vi "DMSP_add_NaOH_BM.vi"(6 "COM Port":refnum<visa-resource-name>="COM4", 7 "Pump Parameters":T1={"Speed 1"="100", "Speed 2"="250", "Speed 3"="350", "Speed 4"="250", "UW/Sample"="5", "Sparge"="2", "Std"="4", "Waste"="15", "Air"="14", "Milli-Q"="1", "H2SO4"="6", "NaOH"="3", "Catalyst"="7", "Cell (H+ side)"="8", "Cell (sample side)"="9", "NaCl"="11"}, 8 "NaOH Vol (mL)":dbl=3.0, 9 "step to ml":dbl=1920.0, 10 "Total Vol. (mL)":dbl=10.0, 11 "Sample Vol. (mL)":dbl=10.0) -> ()   [LabVIEW 2021]
panel:
  out "Full Command":string="o4A0V5000o1P14400o4D14400o1P33600o4D9600o2D24000o5P9600o2D9600o6P33600o4D33600"
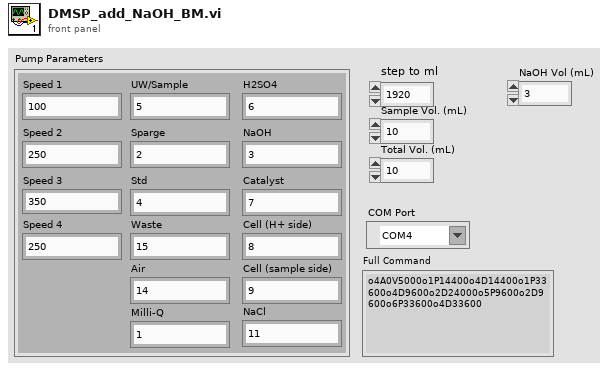
[diagram p1: front panel]
types:
  T1 = cluster{"Speed 1":string, "Speed 2":string, "Speed 3":string, "Speed 4":string, "UW/Sample":string, "Sparge":string, "Std":string, "Waste":string, "Air":string, "Milli-Q":string, "H2SO4":string, "NaOH":string, "Catalyst":string, "Cell (H+ side)":string, "Cell (sample side)":string, "NaCl":string}
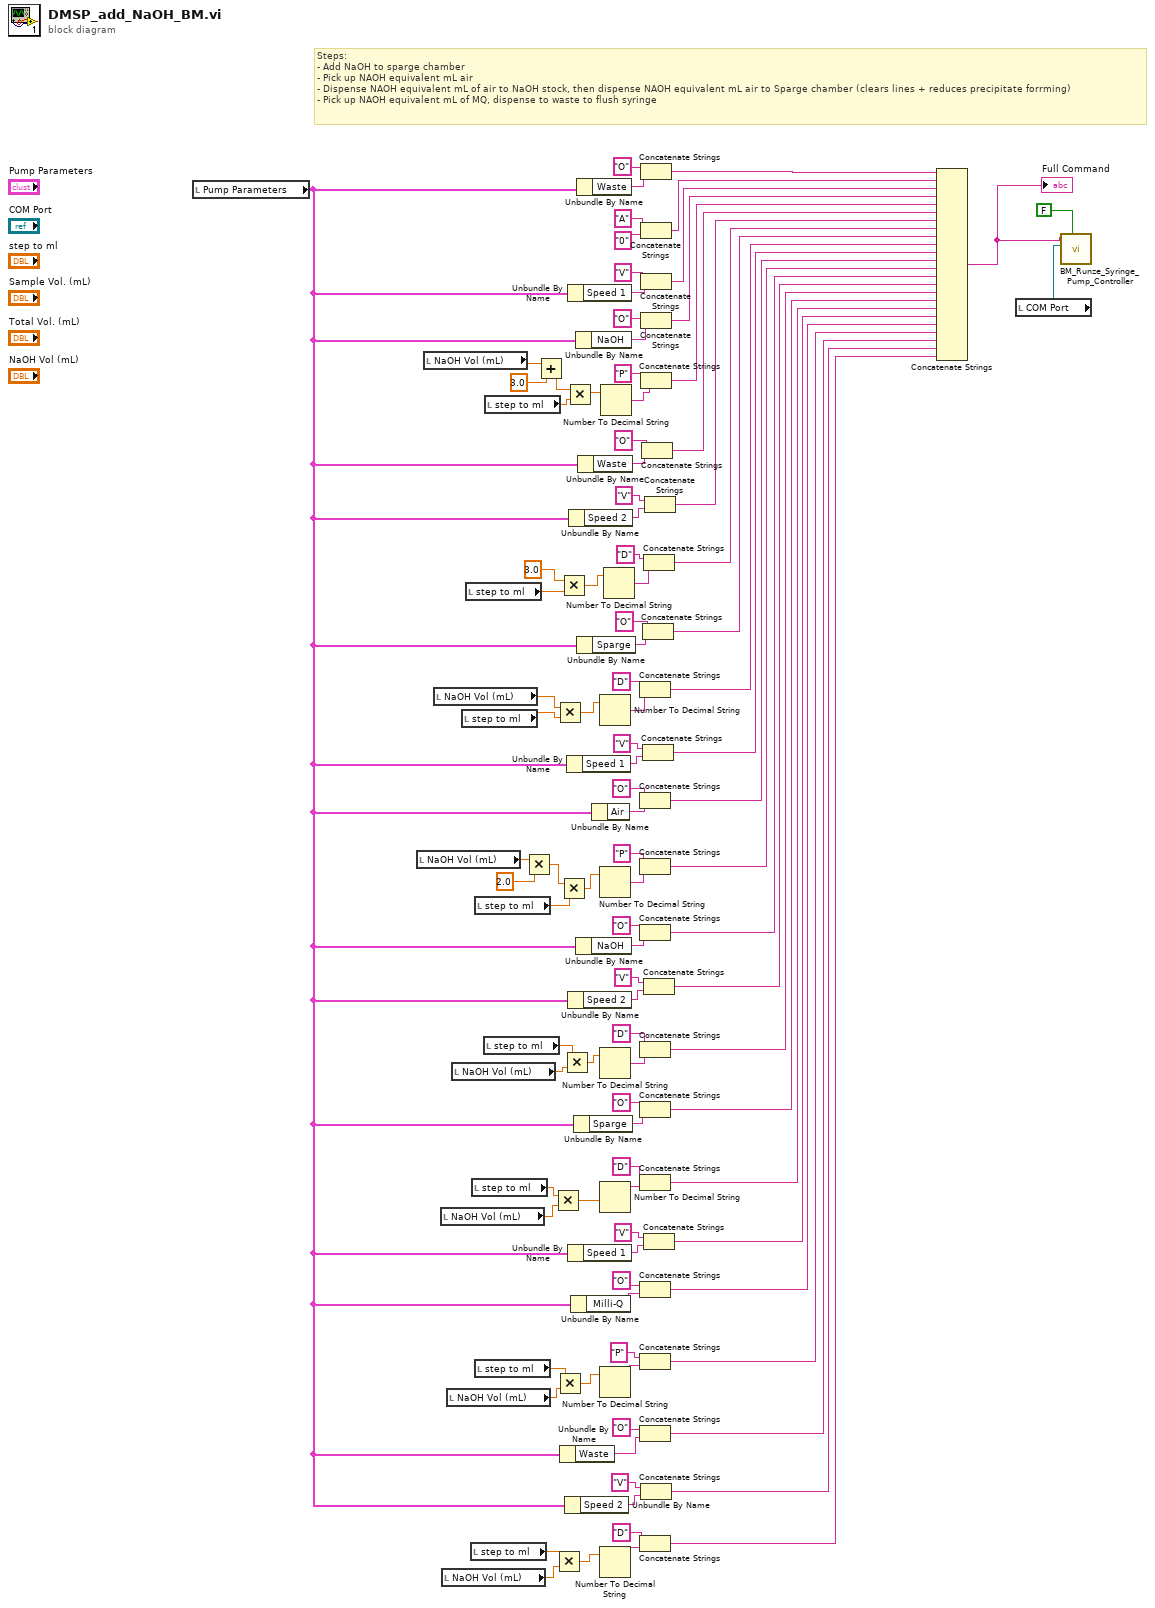
[diagram p0: block diagram]
diagram:
  # "Steps:\n- Add NaOH to sparge chamber\n- Pick up NAOH equivalent mL air \n- Dispense NAOH equivalent mL of air to NaOH stock, then dispense NAOH equivalent mL air to Sparge chamber (clears lines + reduces precipitate forrming)\n- Pick up NAOH equivalent mL of MQ, dispense to waste to flush syringe"
  n1 = local read "Pump Parameters"() -> (w10:T1)
  n2 = local read "NaOH Vol (mL)"() -> (w22:dbl)
  n3 = local read "NaOH Vol (mL)"() -> (w13:dbl)
  n4 = local read "NaOH Vol (mL)"() -> (w23:dbl)
  n5 = local read "NaOH Vol (mL)"() -> (w17:dbl)
  n6 = local read "NaOH Vol (mL)"() -> (w19:dbl)
  n7 = local read "NaOH Vol (mL)"() -> (w18:dbl)
  n8 = local read "NaOH Vol (mL)"() -> (w16:dbl)
  n9 = local read "step to ml"() -> (w71:dbl)
  n10 = local read "step to ml"() -> (w8:dbl)
  n11 = local read "step to ml"() -> (w60:dbl)
  n12 = local read "step to ml"() -> (w85:dbl)
  n13 = local read "step to ml"() -> (w86:dbl)
  n14 = local read "step to ml"() -> (w84:dbl)
  n15 = local read "step to ml"() -> (w87:dbl)
  n16 = local read "step to ml"() -> (w88:dbl)
  n17 = Multiply(x=w22, y=2.0) -> (x*y=w20:dbl)
  n18 = Add(x=w13, y=3.0) -> (x+y=w15:dbl)
  n19 = Multiply(x=w85, y=w17) -> (x*y=w103:dbl)
  n20 = Multiply(x=w60, y=w19) -> (x*y=w61:dbl)
  n21 = Multiply(x=w23, y=w71) -> (x*y=w72:dbl)
  n22 = Multiply(x=w84, y=w18) -> (x*y=w102:dbl)
  n23 = Multiply(x=3.0, y=w8) -> (x*y=w7:dbl)
  n24 = Multiply(x=w20, y=w86) -> (x*y=w101:dbl)
  n25 = Unbundle By Name(w10) -> ("Waste"=w75:string)
  n26 = Multiply(x=w87, y=w16) -> (x*y=w104:dbl)
  n27 = Multiply(x=w15, y=w88) -> (x*y=w100:dbl)
  n28 = Unbundle By Name(w10) -> ("Speed 2"=w46:string)
  n29 = Unbundle By Name(w10) -> ("Speed 1"=w53:string)
  n30 = Unbundle By Name(w10) -> ("Speed 1"=w82:string)
  n31 = Unbundle By Name(w10) -> ("Speed 2"=w50:string)
  n32 = Unbundle By Name(w10) -> ("Speed 1"=w49:string)
  n33 = Unbundle By Name(w10) -> ("Speed 2"=w54:string)
  n34 = Unbundle By Name(w10) -> ("Milli-Q"=w76:string)
  n35 = Unbundle By Name(w10) -> ("Sparge"=w77:string)
  n36 = Unbundle By Name(w10) -> ("NaOH"=w81:string)
  n37 = Unbundle By Name(w10) -> ("NaOH"=w78:string)
  n38 = Unbundle By Name(w10) -> ("Waste"=w83:string)
  n39 = Unbundle By Name(w10) -> ("Sparge"=w80:string)
  n40 = Unbundle By Name(w10) -> ("Waste"=w12:string)
  n41 = Unbundle By Name(w10) -> ("Air"=w79:string)
  n42 = Number To Decimal String(number=w72) -> (decimal integer string=w69:string)  [unwired: 1 out]
  n43 = Number To Decimal String(number=w101) -> (decimal integer string=w67:string)  [unwired: 1 out]
  n44 = Number To Decimal String(number=w104) -> (decimal integer string=w66:string)  [unwired: 1 out]
  n45 = Number To Decimal String(number=w103) -> (decimal integer string=w63:string)  [unwired: 1 out]
  n46 = Number To Decimal String(number=w102) -> (decimal integer string=w59:string)  [unwired: 1 out]
  n47 = Number To Decimal String(number=w61) -> (decimal integer string=w57:string)  [unwired: 1 out]
  n48 = Number To Decimal String(number=w100) -> (decimal integer string=w70:string)  [unwired: 1 out]
  n49 = Number To Decimal String(number=w7) -> (decimal integer string=w9:string)  [unwired: 1 out]
  n50 = Concatenate Strings("D", w69) -> (w39:string)
  n51 = Concatenate Strings("O", w79) -> (w37:string)
  n52 = Concatenate Strings("P", w67) -> (w36:string)
  n53 = Concatenate Strings("O", w78) -> (w35:string)
  n54 = Concatenate Strings("D", w66) -> (w33:string)
  n55 = Concatenate Strings("O", w77) -> (w32:string)
  n56 = Concatenate Strings("D", w63) -> (w31:string)
  n57 = Concatenate Strings("O", w76) -> (w29:string)
  n58 = Concatenate Strings("P", w59) -> (w28:string)
  n59 = Concatenate Strings("O", w75) -> (w27:string)
  n60 = Concatenate Strings("D", w57) -> (w25:string)
  n61 = Concatenate Strings("O", w83) -> (w44:string)
  n62 = Concatenate Strings("A", "0") -> (w43:string)
  n63 = Concatenate Strings("V", w82) -> (w42:string)
  n64 = Concatenate Strings("O", w81) -> (w41:string)
  n65 = Concatenate Strings("P", w70) -> (w40:string)
  n66 = Concatenate Strings("V", w46) -> (w26:string)
  n67 = Concatenate Strings("O", w12) -> (w4:string)
  n68 = Concatenate Strings("O", w80) -> (w3:string)
  n69 = Concatenate Strings("V", w53) -> (w38:string)
  n70 = Concatenate Strings("D", w9) -> (w2:string)
  n71 = Concatenate Strings("V", w50) -> (w34:string)
  n72 = Concatenate Strings("V", w49) -> (w30:string)
  n73 = Concatenate Strings("V", w54) -> (w1:string)
  n74 = Concatenate Strings(w44, w43, w42, w41, w40, w4, w1, w2, w3, w39, w38, w37, w36, w35, w34, w33, w32, w31, w30, w29, w28, w27, w26, w25) -> (w91:string)
  "Full Command" <- w91
  n75 = local read "COM Port"() -> (w90:refnum<visa-resource-name>)
  n76 = call "BM_Runze_Syringe_Pump_Controller.vi"("Initialize Plunger?"=FALSE ("Initialize?"), "COM Port (Runze)"=w90, "Enter Command"=w91) -> ()  [unwired: 6 in, 3 out]
